vi "mainVI.vi"() -> ()   [LabVIEW 2024]
uses:
  controls/#typedef_Waveform_Type.ctl
  controls/#typedef_Data_Cluster.ctl
  <vilib>/sound2/lvsound2.llb/Sound Data Format.ctl
  <vilib>/sound2/lvsound2.llb/Sound Output Task ID.ctl
  controls/#typedef_StateMachine_States.ctl
  <vilib>/sound2/lvsound2.llb/Sampling Mode.ctl
  <vilib>/Analysis/4window.llb/windowTd.ctl
  <vilib>/numeric/Random Number (Range) DBL.vi
  <vilib>/measure/maspectr.llb/FFT Power Spectrum and PSD for 1 Chan.vi
  <vilib>/sound2/lvsound2.llb/Sound Output Write (DBL Single).vi
  <vilib>/Analysis/NI_AALBase.lvlib
  <vilib>/measure/NI_MAPro.lvlib
  <vilib>/Analysis/NI_AALPro.lvlib
panel:
  out "Waveform":waveform(dbl)
  out "error out":errorcluster
  in  "Volume":dbl(knob) scale=0.0..1.0
  out "FFT Graph":cluster{"f0":dbl, "df":dbl, "magnitude":dbl[]}(graph)
  out "Waveform Graph":waveform(dbl)(graph)
  out "XY Graph":cluster{dbl[], dbl[]}(graph)
  in  "Attack":i32(slide) scale=1.0..100.0
  in  "Release":i32(slide) scale=1.0..100.0
  out "Main Data Cluster":T1={"Notes Frequency Array"=[], "Waveform Type"=enum."Sine", "Waveform"={"t0"=timestamp(0 s since 1904-01-01), "dt"=1.0, "Y"=[]}, "Current Note"=0, "Octave Range Offset"=0, "sound format"={"sample rate (S/s)"=22050.0, "number of channels"=2, "bits per sample"=16}, "Task ID"=0, "Note Duration"=0.0, "Release Env"=0, "Attack Env"=0, "Volume"=0.0} {"task ID" format="%.0x"}
  in  "device ID":u32
  in  "OK Button":bool
  in  "Settings Button":bool
  in  "Octave Range":u32(knob)=2 max=5 step=1 scale=0.0..5.0
  in  "Waveform Type":T2
  in  "BPM":dbl(knob) scale=0.1..1.0
  in  "Dial 12":dbl(knob) scale=0.0..12.0
  in  "Dial 16":dbl(knob) scale=0.0..12.0
  in  "Dial 15":dbl(knob) scale=0.0..12.0
  in  "Dial 14":dbl(knob) scale=0.0..12.0
  in  "Dial 11":dbl(knob) scale=0.0..12.0
  in  "Dial 13":dbl(knob) scale=0.0..12.0
  in  "Dial 10":dbl(knob) scale=0.0..12.0
  in  "Dial 9":dbl(knob) scale=0.0..12.0
  in  "Dial 8":dbl(knob) scale=0.0..12.0
  in  "Dial 7":dbl(knob) scale=0.0..12.0
  in  "Dial 6":dbl(knob) scale=0.0..12.0
  in  "Dial 5":dbl(knob) scale=0.0..12.0
  in  "Dial 4":dbl(knob) scale=0.0..12.0
  in  "Dial 3":dbl(knob) scale=0.0..12.0
  in  "Dial 2":dbl(knob) scale=0.0..12.0
  in  "Dial 1":dbl(knob)=1.0 min=1.0 step=1.0 scale=0.0..12.0
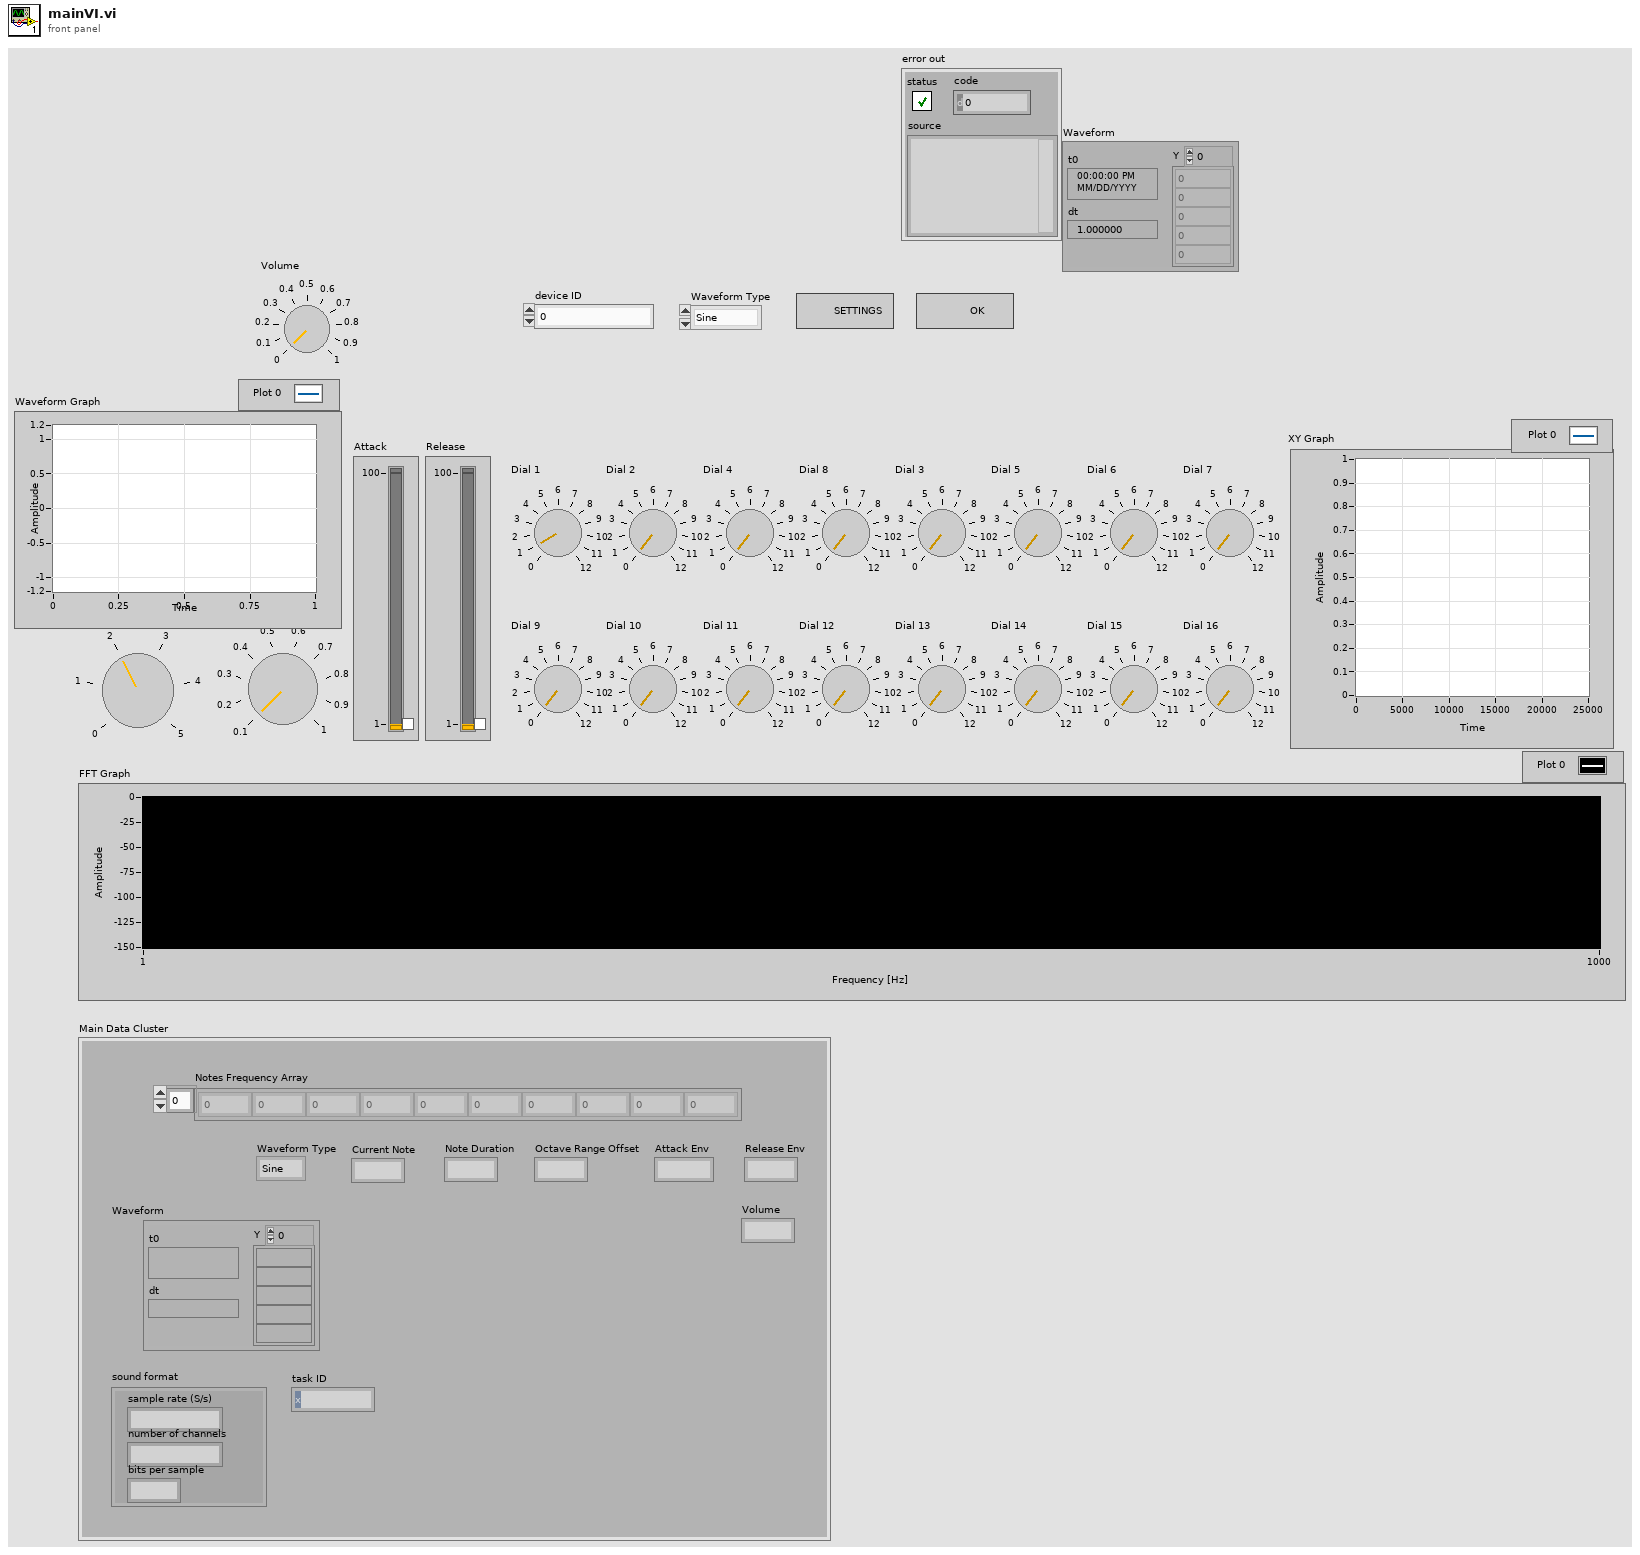
[diagram p1: front panel]
types:
  T1 = typedef "#typedef_Data_Cluster.ctl" = cluster{"Notes Frequency Array":dbl[], "Waveform Type":T2, "Waveform":waveform(dbl), "Current Note":i32, "Octave Range Offset":u32, "sound format":T3, "Task ID":T4, "Note Duration":dbl, "Release Env":i32, "Attack Env":i32, "Volume":dbl}
  T2 = typedef "#typedef_Waveform_Type.ctl" = enum16{"Sine", "Saw", "Square", "Triangle", "Noise"}
  T3 = typedef "Sound Data Format.ctl" = cluster{"sample rate (S/s)":dbl, "number of channels":i32, "bits per sample":i32}
  T4 = typedef "Sound Output Task ID.ctl" = u32
  T5 = typedef "#typedef_StateMachine_States.ctl" = enum16{"Stop", "Init", "Idle", "Settings", "Write Data", "Read Data", "Play Data", "Err"}
  T6 = typedef "Sampling Mode.ctl" = i32
  T7 = typedef "NI_AALPro.lvlib/windowTd.ctl" = u32
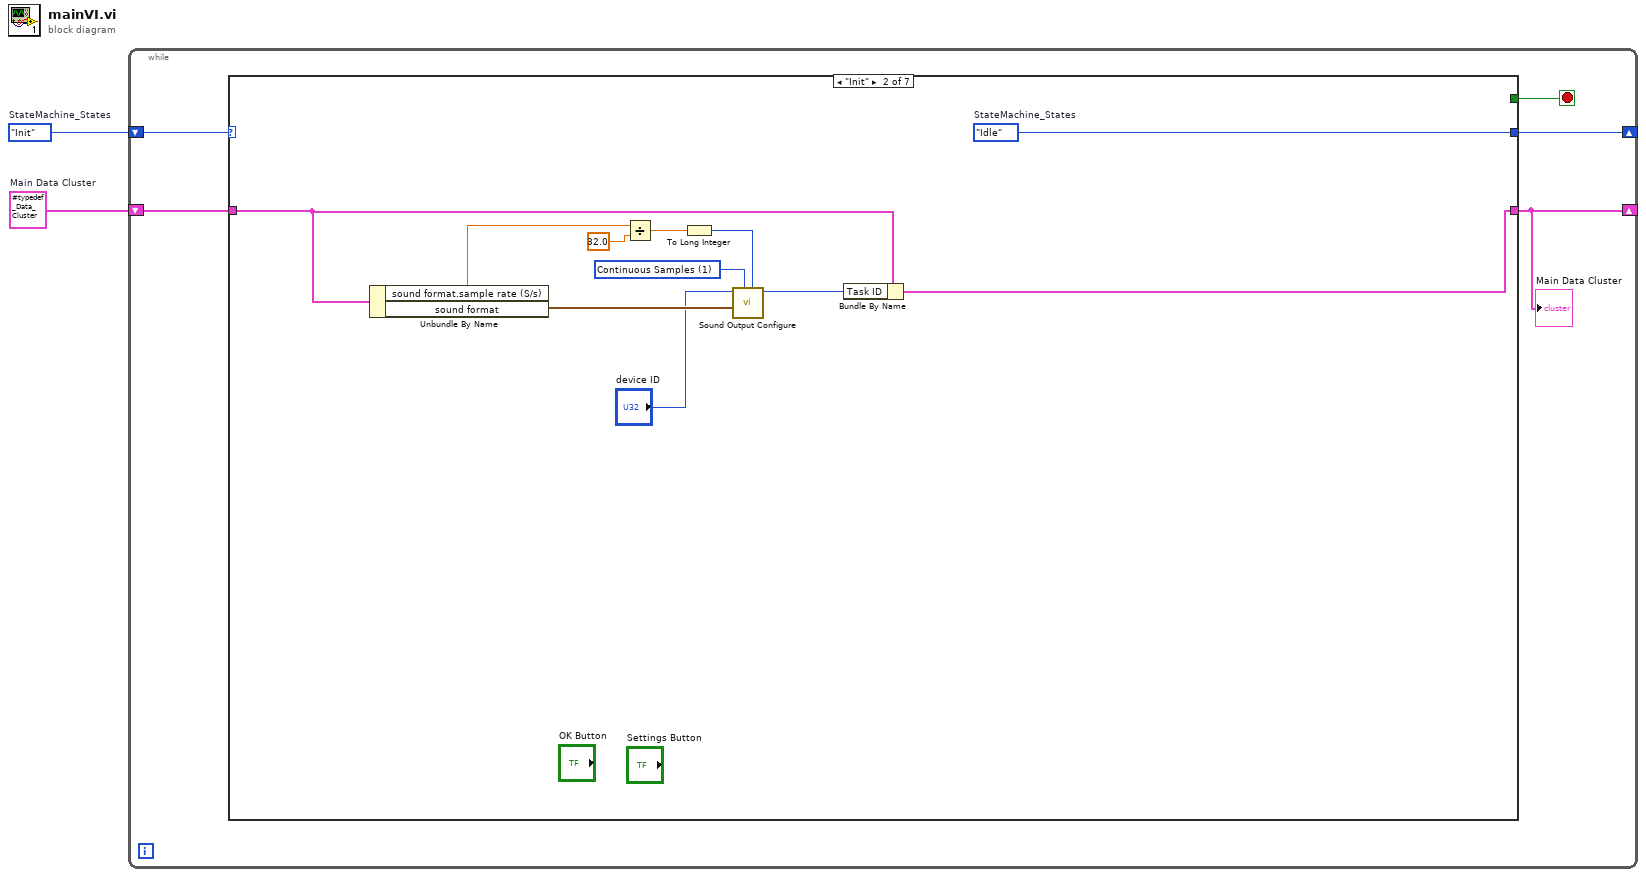
[diagram p0: block diagram]
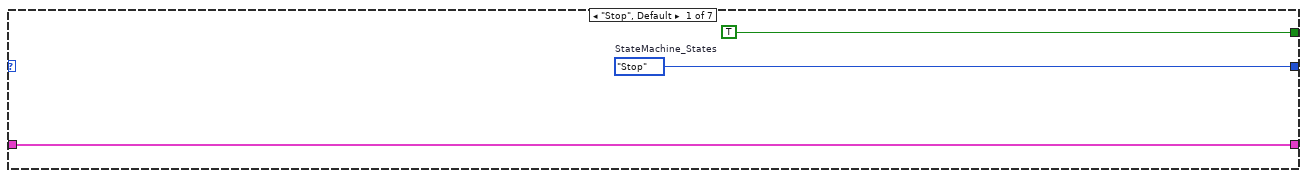
[diagram p2: hidden frame]
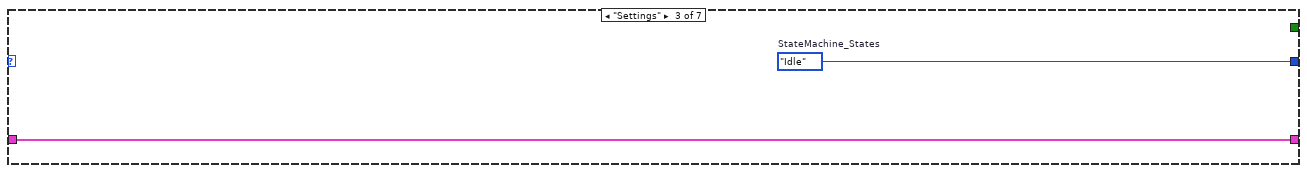
[diagram p3: hidden frame]
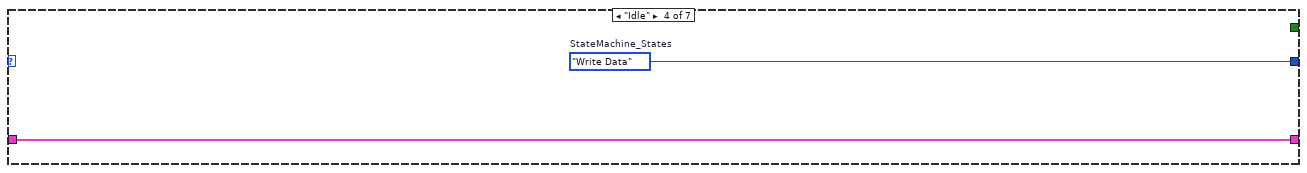
[diagram p4: hidden frame]
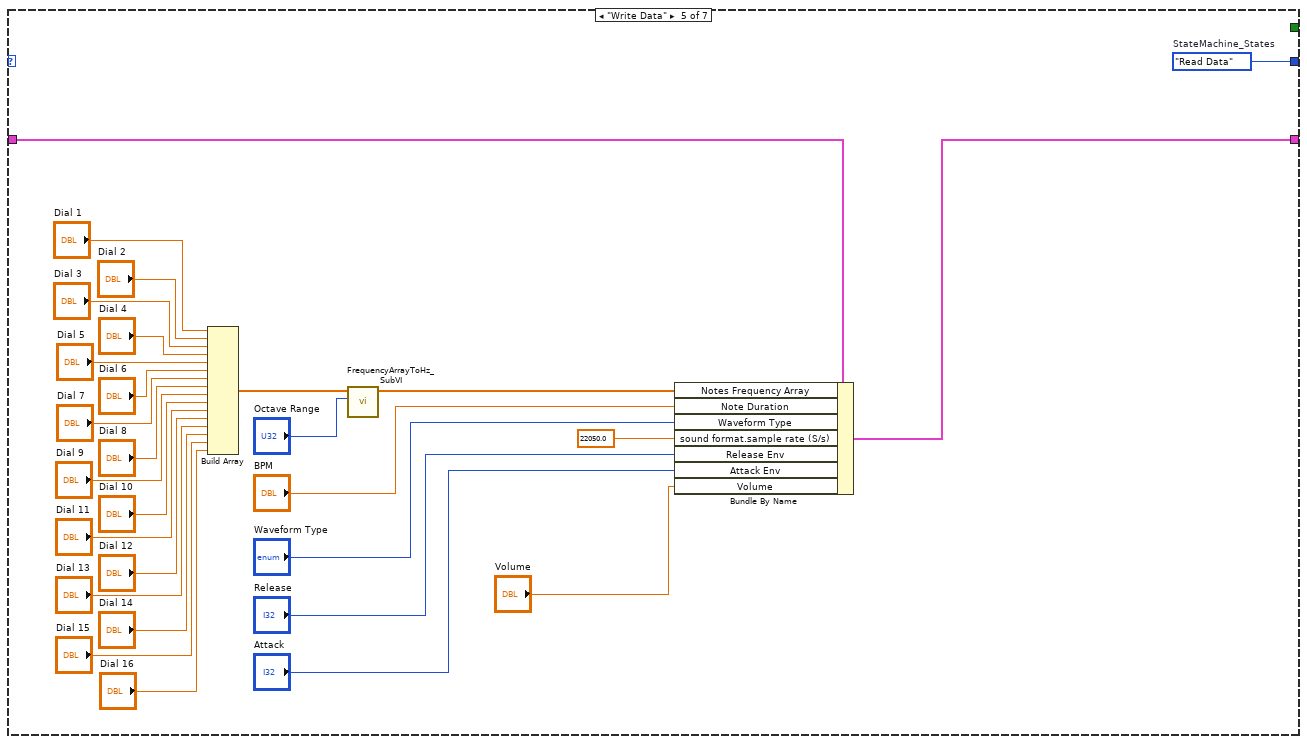
[diagram p5: hidden frame]
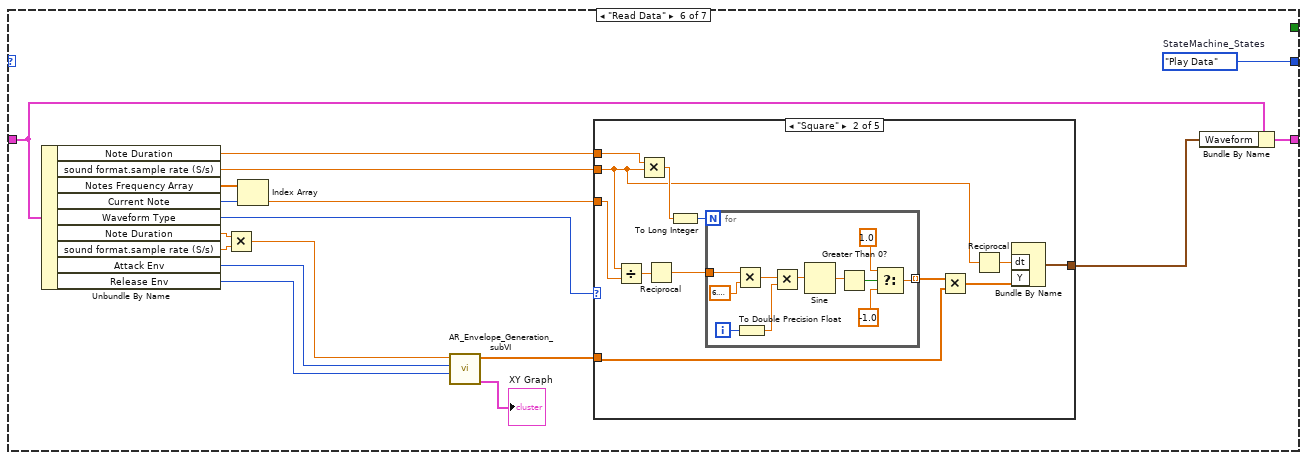
[diagram p6: hidden frame]
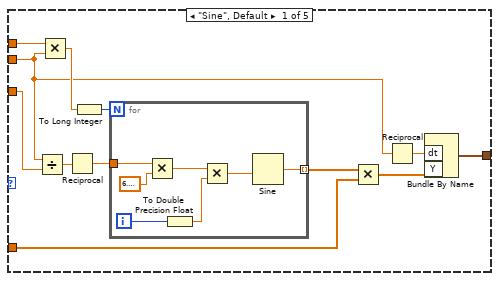
[diagram p7: hidden frame]
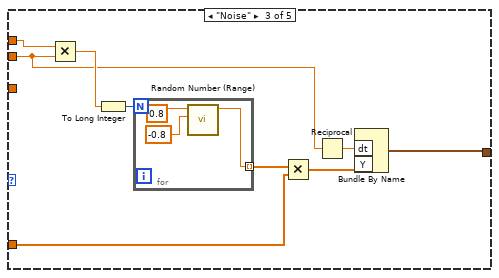
[diagram p8: hidden frame]
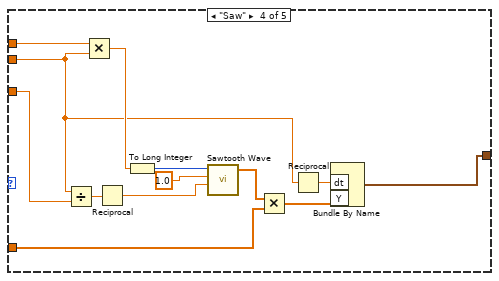
[diagram p9: hidden frame]
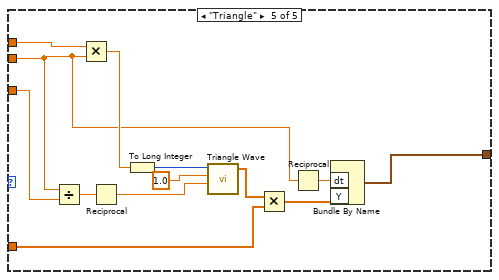
[diagram p10: hidden frame]
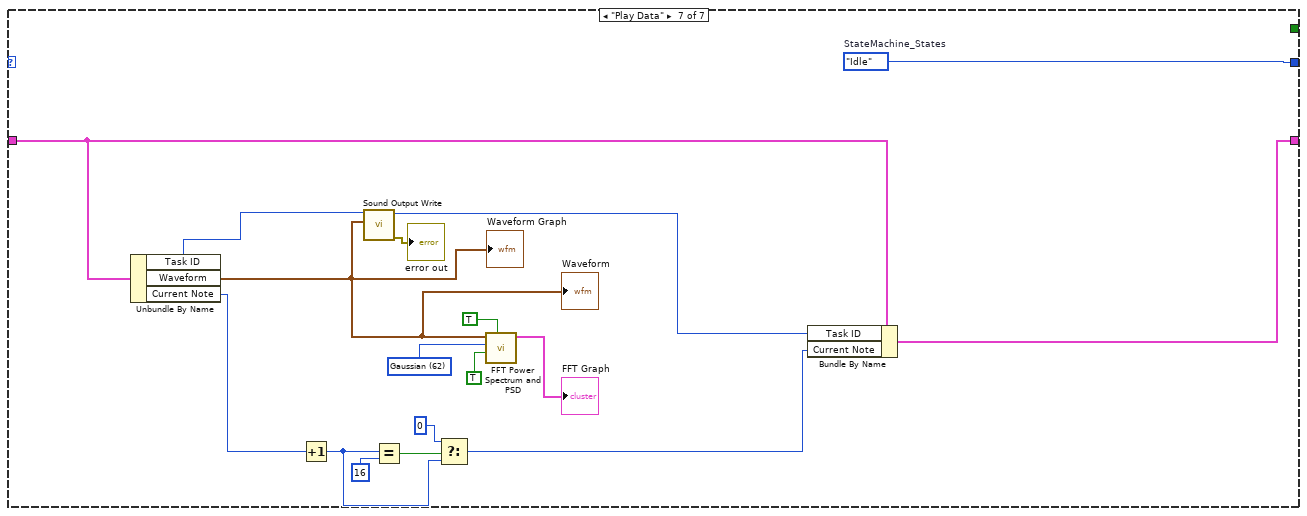
[diagram p11: hidden frame]
diagram:
  w1 = T1 {"Notes Frequency Array"=[], "Waveform Type"=enum."Sine", "Waveform"={"t0"=timestamp(0 s since 1904-01-01), "dt"=1.0, "Y"=[]}, "Current Note"=0, "Octave Range Offset"=0, "sound format"={"sample rate (S/s)"=22050.0, "number of channels"=2, "bits per sample"=16}, "Task ID"=0, "Note Duration"=0.0, "Release Env"=0, "Attack Env"=0, "Volume"=0.0}  # Main Data Cluster
  w2 = #typedef_StateMachine_States."Init"  # StateMachine_States
  n1 = while {
    shift-right: [w6] -> _
    shift-left: w2 -> [w7]
    shift-right: [w3] -> _
    shift-left: w1 -> [w4]
    stop <- w5 stop-if-true
    n2 = case shown="\"Init\"" w7 {
      tunnel: [w10 w21 w23 w25 w35 w66 w167] -> w6
      tunnel: [TRUE _ _ _ _ _ _] -> w5
      tunnel: w4 -> [w8 w13 w22 w24 w37 w65 w161]
      tunnel: [w8 w12 w22 w24 w31 w68 w159] -> w3
      frame "Stop", Default {
        w10 = #typedef_StateMachine_States."Stop"  # StateMachine_States
      }
      frame "Init" {
        w20 = T6 1 items=["Finite Samples", "Continuous Samples"] ("sample mode")
        w21 = #typedef_StateMachine_States."Idle"  # StateMachine_States
        n3 = Unbundle By Name(w13) -> ("sound format.sample rate (S/s)"=w18:dbl, "sound format"=w19:T3)
        n4 = Divide(x=w18, y=32.0) -> (x/y=w17:dbl)
        n5 = To Long Integer(number=w17) -> (32bit integer=w15:i32)
        n6 = call <vilib>:"Sound Output Configure.vi"("number of samples/ch"=w15, "sample mode"=w20, "sound format"=w19, "device ID"="device ID") -> ("task ID"=w14:T4)  [unwired: 6 in, 1 out]
        n7 = Bundle By Name(cluster=w13, "Task ID"=w14) -> (w12:T1)
      }
      frame "Settings" {
        w23 = #typedef_StateMachine_States."Idle"  # StateMachine_States
      }
      frame "Idle" {
        w25 = #typedef_StateMachine_States."Write Data"  # StateMachine_States
      }
      frame "Write Data" {
        w35 = #typedef_StateMachine_States."Read Data"  # StateMachine_States
        n8 = Build Array("Dial 1", "Dial 2", "Dial 3", "Dial 4", "Dial 5", "Dial 6", "Dial 7", "Dial 8", "Dial 9", "Dial 10", "Dial 11", "Dial 12", "Dial 13", "Dial 14", "Dial 15", "Dial 16") -> (w34:dbl[])
        n9 = call "FrequencyArrayToHz_SubVI.vi"("Octave Range in"="Octave Range", "Notes array in"=w34) -> ("Frequency array out"=w30:dbl[])  [unwired: 9 in]
        n10 = Bundle By Name(cluster=w37, "Notes Frequency Array"=w30, "Note Duration"="BPM", "Waveform Type"="Waveform Type", "sound format.sample rate (S/s)"=22050.0, "Release Env"="Release", "Attack Env"="Attack", "Volume"="Volume") -> (w31:T1)
      }
      frame "Read Data" {
        w66 = #typedef_StateMachine_States."Play Data"  # StateMachine_States
        n11 = Unbundle By Name(w65) -> ("Note Duration"=w61:dbl, "sound format.sample rate (S/s)"=w62:dbl, "Notes Frequency Array"=w69:dbl[], "Current Note"=w63:i32, "Waveform Type"=w70:T2, "Note Duration"=w58:dbl, "sound format.sample rate (S/s)"=w59:dbl, "Attack Env"=w56:i32, "Release Env"=w57:i32)
        n12 = Multiply(x=w58, y=w59) -> (x*y=w60:dbl)
        n13 = Index Array(array=w69, index=w63) -> (element=w64:dbl)
        n14 = call "AR_Envelope_Generation_subVI.vi"("Release in"=w57, "Attack  in"=w56, "Number of Samples in"=w60) -> ("Envelope XY Graph out"=→"XY Graph":cluster{dbl[], dbl[]}, "Envelope Array out"=w54:dbl[])  [unwired: 7 in]
        n15 = case shown="\"Square\"" w70 {
          tunnel: w64 -> [w80 w99 _ w134 w145]
          tunnel: w62 -> [w71 w90 w113 w125 w138]
          tunnel: [w78 w91 w114 w126 w139] -> w67
          tunnel: w61 -> [w76 w97 w120 w135 w148]
          tunnel: w54 -> [w74 w92 w115 w129 w142]
          frame "Sine", Default {
            n16 = Divide(x=w71, y=w80) -> (x/y=w81:dbl)
            n17 = Multiply(x=w76, y=w71) -> (x*y=w75:dbl)
            n18 = Reciprocal(x=w81) -> (1/x=w79:dbl)
            n19 = To Long Integer(number=w75) -> (32bit integer=w82:i32)
            n20 = for {
              N: w82 -> [_]
              tunnel: w79 -> [w89]
              tunnel: [w87] -> w73 mode=indexing
              i -> [w84]
              n21 = Multiply(x=w89, y=6.283185307179586) -> (x*y=w86:dbl)
              n22 = To Double Precision Float(number=w84) -> (double precision float=w83:dbl)
              n23 = Multiply(x=w86, y=w83) -> (x*y=w85:dbl)
              n24 = Sine(x=w85) -> (sin(x)=w87:dbl)
            }
            n25 = Multiply(x=w73, y=w74) -> (x*y=w72:dbl[])
            n26 = Reciprocal(x=w71) -> (1/x=w77:dbl)
            n27 = Bundle By Name("dt"=w77, "Y"=w72) -> (w78:waveform(dbl))  [unwired: 1 in]
          }
          frame "Square" {
            n28 = Divide(x=w90, y=w99) -> (x/y=w100:dbl)
            n29 = Multiply(x=w97, y=w90) -> (x*y=w95:dbl)
            n30 = Reciprocal(x=w100) -> (1/x=w98:dbl)
            n31 = To Long Integer(number=w95) -> (32bit integer=w101:i32)
            n32 = for {
              N: w101 -> [_]
              tunnel: w98 -> [w112]
              tunnel: [w106] -> w93 mode=indexing
              i -> [w103]
              n33 = Multiply(x=w112, y=6.283185307179586) -> (x*y=w104:dbl)
              n34 = To Double Precision Float(number=w103) -> (double precision float=w102:dbl)
              n35 = Multiply(x=w104, y=w102) -> (x*y=w105:dbl)
              n36 = Sine(x=w105) -> (sin(x)=w107:dbl)
              n37 = Greater Than 0?(x=w107) -> (x > 0?=w110:bool)
              n38 = Select(t=1.0, s=w110, f=-1.0) -> (s? t:f=w106:dbl)
            }
            n39 = Multiply(x=w93, y=w92) -> (x*y=w94:dbl[])
            n40 = Reciprocal(x=w90) -> (1/x=w96:dbl)
            n41 = Bundle By Name("dt"=w96, "Y"=w94) -> (w91:waveform(dbl))  [unwired: 1 in]
          }
          frame "Noise" {
            n42 = Multiply(x=w120, y=w113) -> (x*y=w117:dbl)
            n43 = To Long Integer(number=w117) -> (32bit integer=w121:i32)
            n44 = for {
              N: w121 -> [_]
              tunnel: [w122] -> w116 mode=indexing
              n45 = call-poly <vilib>:"Random Number (Range).vi"("lower bound (0)"=-0.8, "upper bound (100)"=0.8) -> ("number"=w122:dbl)  [unwired: 9 in]
            }
            n46 = Multiply(x=w116, y=w115) -> (x*y=w118:dbl[])
            n47 = Reciprocal(x=w113) -> (1/x=w119:dbl)
            n48 = Bundle By Name("dt"=w119, "Y"=w118) -> (w114:waveform(dbl))  [unwired: 1 in]
          }
          frame "Saw" {
            n49 = Divide(x=w125, y=w134) -> (x/y=w133:dbl)
            n50 = Multiply(x=w135, y=w125) -> (x*y=w127:dbl)
            n51 = Reciprocal(x=w133) -> (1/x=w132:dbl)
            n52 = To Long Integer(number=w127) -> (32bit integer=w136:i32)
            n53 = call <vilib>:"Sawtooth Wave.vi"("samples"=w136, "amplitude"=1.0, "frequency"=w132) -> ("sawtooth wave"=w128:dbl[])  [unwired: 2 in, 2 out]
            n54 = Multiply(x=w128, y=w129) -> (x*y=w130:dbl[])
            n55 = Reciprocal(x=w125) -> (1/x=w131:dbl)
            n56 = Bundle By Name("dt"=w131, "Y"=w130) -> (w126:waveform(dbl))  [unwired: 1 in]
          }
          frame "Triangle" {
            n57 = Divide(x=w138, y=w145) -> (x/y=w146:dbl)
            n58 = Multiply(x=w148, y=w138) -> (x*y=w140:dbl)
            n59 = Reciprocal(x=w146) -> (1/x=w147:dbl)
            n60 = To Long Integer(number=w140) -> (32bit integer=w149:i32)
            n61 = call <vilib>:"Triangle Wave.vi"("samples"=w149, "amplitude"=1.0, "frequency"=w147) -> ("triangle wave"=w141:dbl[])  [unwired: 2 in, 2 out]
            n62 = Multiply(x=w141, y=w142) -> (x*y=w143:dbl[])
            n63 = Reciprocal(x=w138) -> (1/x=w144:dbl)
            n64 = Bundle By Name("dt"=w144, "Y"=w143) -> (w139:waveform(dbl))  [unwired: 1 in]
          }
        }
        n65 = Bundle By Name(cluster=w65, "Waveform"=w67) -> (w68:T1)
      }
      frame "Play Data" {
        w156 = T7 62 items=["Rectangle"=0, "Hanning"=1, "Hamming"=2, "Blackman-Harris"=3, "Exact Blackman"=4, "Blackman"=5, "Flat Top"=6, "4 Term B-Harris "=7, "7 Term B-Harris"=8, "Low Sidelobe"=9, "Blackman Nuttall"=11, "Triangle"=30, "Bartlett-Hanning"=31, "Bohman"=32, "Parzen"=33, "Welch"=34, "Kaiser"=60, "Dolph-Chebyshev"=61, "Gaussian"=62] ("window")
        w167 = #typedef_StateMachine_States."Idle"  # StateMachine_States
        n66 = Unbundle By Name(w161) -> ("Task ID"=w158:T4, "Waveform"=w151:waveform(dbl), "Current Note"=w166:i32)
        "Waveform Graph" <- w151
        "Waveform" <- w151
        n67 = Increment(x=w166) -> (x+1=w163:i32)
        n68 = call-poly <vilib>:"Sound Output Write.vi"("data"=w151, "task ID"=w158) -> ("error out"=→"error out":errorcluster, "task ID out"=w157:T4)  [unwired: 8 in]
        n69 = Equal?(x=w163, y=16) -> (x = y?=w164:bool)
        n70 = Select(t=0, s=w164, f=w163) -> (s? t:f=w160:i32)
        n71 = call-poly <vilib>:"FFT Power Spectrum and PSD.vi"("restart averaging (F)"=TRUE, "dB On (F)"=TRUE, "window"=w156, "time signal"=w151) -> ("Power Spectrum / PSD"=→"FFT Graph":cluster{"f0":dbl, "df":dbl, "magnitude":dbl[]})  [unwired: 4 in, 3 out]
        n72 = Bundle By Name(cluster=w161, "Task ID"=w157, "Current Note"=w160) -> (w159:T1)
      }
    }
    "Main Data Cluster" <- w3
  }
